vi "Untitled 3 (SubVI).vi"(0 "Refnum in":T1, 1 "LapTop Cam":bool, 2 "Vision":u16, 5 "New Image in":T1, 7 "Camera IP":string, 9 "Rec Mode":enum32{"Stop", "Record", "Playback"}(ring), 11 "Show Black And White":bool, 12 "LED Color":T3, 13 "Camera Settings":T2) -> (3 "Bandwidth (Mbps)":dbl, 4 "Refnum out":T1, 6 "Array":cluster{"Color Box":u32, "Color Box":u32}[](array[cluster]), 8 "Numeric 2":dbl, 10 "Numeric":dbl, 14 "FPS":dbl, 15 "status":bool)   [LabVIEW 2015]
uses:
  <vilib>/vision/Image Controls.llb/IMAQ Image.ctl
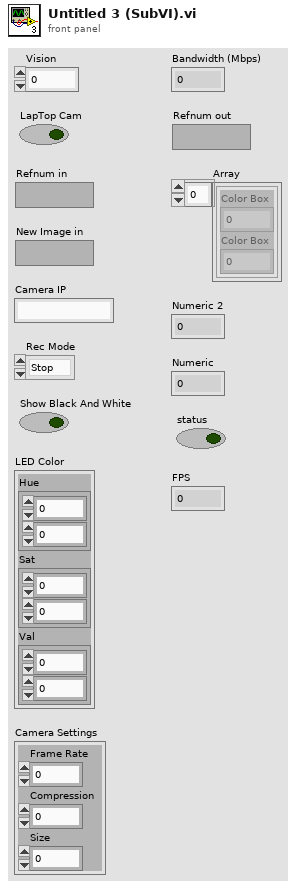
[diagram p1: front panel]
types:
  T1 = typedef "IMAQ Image.ctl" = refnum<image>
  T2 = cluster{"Frame Rate":i32, "Compression":i32, "Size":u16}
  T3 = cluster{"Hue":cluster{dbl, dbl}, "Sat":cluster{dbl, dbl}, "Val":cluster{dbl, dbl}}
  T4 = cluster{"Distance (ft)":dbl, "Center":cluster{dbl, dbl}, "Normalized Rect":cluster{"Numeric":dbl, "Numeric 2":dbl, "Numeric 3":dbl, "Numeric 5":dbl}}[]
  T5 = cluster{"Distance (ft)":dbl, "Center":cluster{dbl, dbl}, "Normalized Rect":cluster{"Numeric":dbl, "Numeric 2":dbl, "Numeric 3":dbl, "Numeric 5":dbl}}
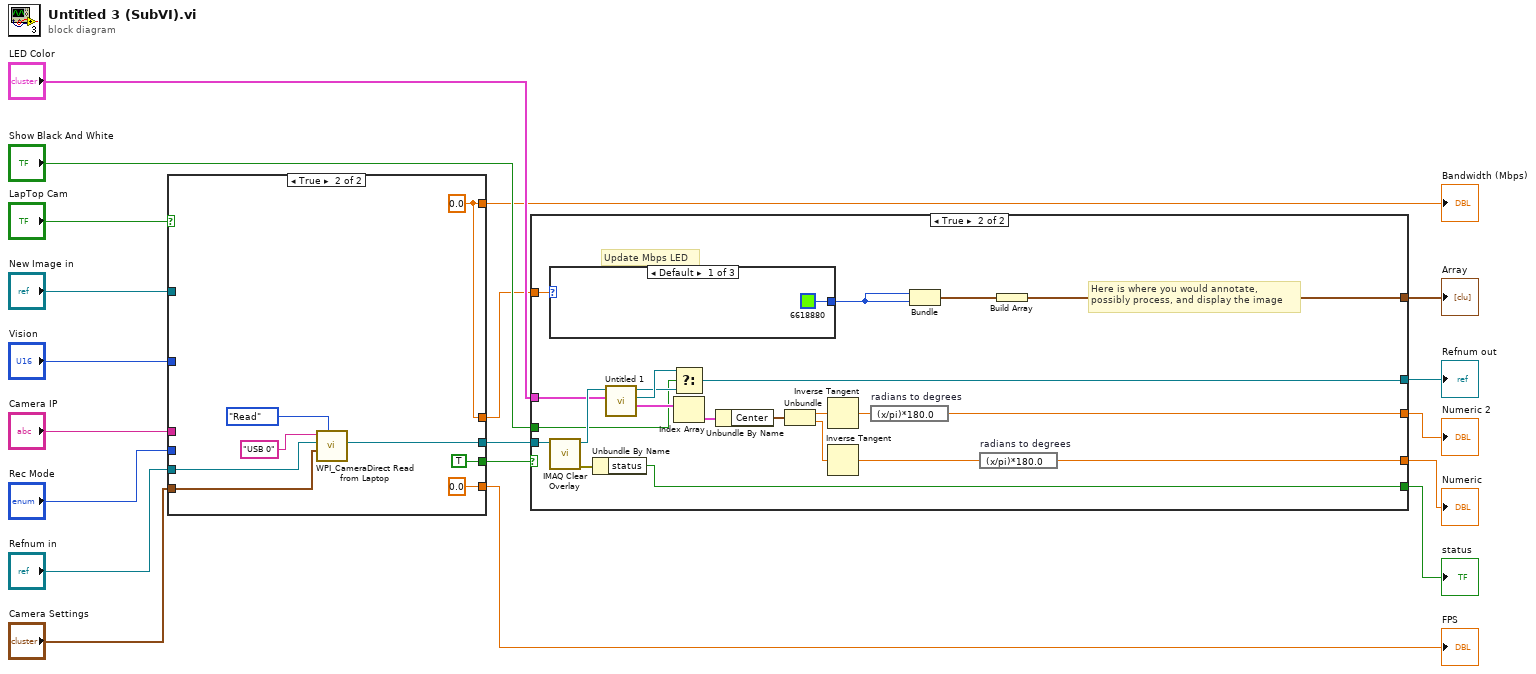
[diagram p0: block diagram]
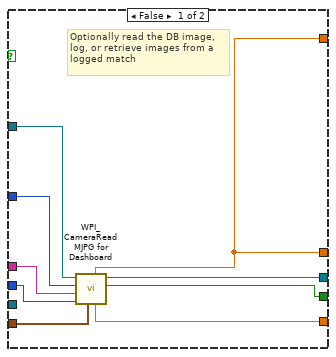
[diagram p2: hidden frame]
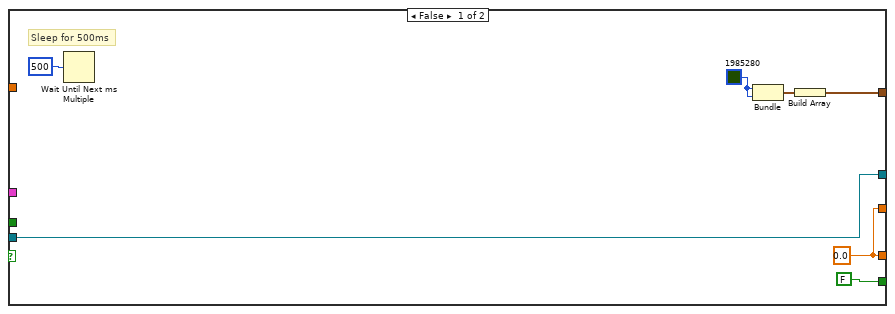
[diagram p3: hidden frame]
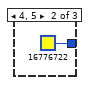
[diagram p4: hidden frame]
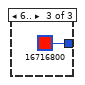
[diagram p5: hidden frame]
diagram:
  n1 = case shown="True" "LapTop Cam" {
    tunnel: "New Image in" -> [w28 _]
    tunnel: [w27 w30] -> w2
    tunnel: [w26 TRUE ("Active")] -> w3
    tunnel: [w25 0.0 ("FPS")] -> w12
    tunnel: [w21 w34] -> w4
    tunnel: "Refnum in" -> [_ w31]
    tunnel: "Camera Settings" -> [w24 w29]
    tunnel: "Camera IP" -> [w23 _]
    tunnel: "Vision" -> [w22 _]
    tunnel: [w21 w34] -> w10
    tunnel: "Rec Mode" -> [w20 _]
    frame False {
      # "Optionally read the DB image,\nlog, or retrieve images from a\nlogged match"
      n2 = call <vilib>:"WPI_CameraRead MJPG for Dashboard.vi"("Camera Settings"=w24, "Rec Mode"=w20, "Camera IP"=w23, "Camera Mode"=w22, "Refnum in"=w28) -> ("Active"=w26:bool, "Refnum out"=w27:T1, "FPS"=w25:dbl, "Bandwidth (Mbps)"=w21:dbl)  [unwired: 3 in]
    }
    frame True {
      w34 = 0.0 ("Bandwidth (Mbps)")
      n3 = call <vilib>:"WPI_CameraDirect Read from Laptop.vi"("Operation"=enum16{"Read", "Reopen", "Close"}."Read", "Camera Settings"=w29, "Image"=w31, "address"="USB 0") -> ("Image Out"=w30:T1)  [unwired: 6 in, 1 out]
    }
  }
  "FPS" <- w12
  "Bandwidth (Mbps)" <- w10
  n4 = case shown="True" w3 {
    tunnel: w2 -> [w39 w62]
    tunnel: w4 -> [_ w61]
    tunnel: [w40 w50] -> w13
    tunnel: [w39 w49] -> w14
    tunnel: [w38 w48] -> w15
    tunnel: [w38 w47] -> w16
    tunnel: [FALSE ("status") w46] -> w17
    tunnel: "LED Color" -> [_ w45]
    tunnel: "Show Black And White" -> [_ w44]
    frame False {
      w38 = 0.0
      w41 = u32 1985280 ("Color Box")
      # "Sleep for 500ms"
      n5 = Wait Until Next ms Multiple(millisecond multiple=u32 500) -> ()  [unwired: 1 out]
      n6 = Bundle("Color Box"=w41, "Color Box"=w41) -> (w42:cluster{"Color Box":u32, "Color Box":u32})  [unwired: 1 out]
      n7 = Build Array(w42) -> (w40:cluster{"Color Box":u32, "Color Box":u32}[])
    }
    frame True {
      # "Here is where you would annotate,\npossibly process, and display the image"
      # "Update Mbps LED"
      n8 = case shown="Default" w61 {
        tunnel: [u32 6618880 ("Color Box") u32 16776722 ("Color Box") u32 16716800 ("Color Box")] -> w63
        frame Default {
        }
        frame 4, 5 {
        }
        frame 6.. {
        }
      }
      n9 = call "IMAQ Clear Overlay"("Image"=w62) -> ("error out"=w65:errorcluster, "Image Out"=w60:T1)  [unwired: 2 in, 7 out]
      n10 = Unbundle By Name(w65) -> ("status"=w46:bool)
      n11 = call "Untitled 1.vi"("LED Color"=w45, "New Image"=w60) -> ("Detected Targets"=w59:T4, "Masked"=w52:T1, "Original Image"=w51:T1)  [unwired: 7 in]
      n12 = Select(t=w52, s=w44, f=w51) -> (s? t:f=w49:T1)
      n13 = Index Array(array=w59) -> (element=w58:T5)  [unwired: 1 in]
      n14 = Unbundle By Name(w58) -> ("Center"=w57:cluster{dbl, dbl})
      n15 = Unbundle(w57) -> (w56:dbl, w53:dbl)
      n16 = Inverse Tangent(1:w56) -> (0:w55:dbl)
      n17 = Inverse Tangent(1:w53) -> (0:w54:dbl)
      n18 = expression code="(x/pi)*180.0" "radians to degrees"(w55) -> (w48:dbl)
      n19 = Bundle("Color Box"=w63, "Color Box"=w63) -> (w64:cluster{"Color Box":u32, "Color Box":u32})  [unwired: 1 out]
      n20 = expression code="(x/pi)*180.0" "radians to degrees"(w54) -> (w47:dbl)
      n21 = Build Array(w64) -> (w50:cluster{"Color Box":u32, "Color Box":u32}[])
    }
  }
  "status" <- w17
  "Numeric" <- w16
  "Numeric 2" <- w15
  "Refnum out" <- w14
  "Array" <- w13
